vi "_iWorx - Light & Laser.vi"() -> ()   [LabVIEW 2012]
doc: "This VI is designed to work with myDAQ and the iWorx Light Sensor & Laser x2."
uses:
  <vilib>/DAQmx/create/channels.llb/DAQmx Create Channel (AI-Voltage-Basic).vi
  <vilib>/DAQmx/configure/timing.llb/DAQmx Timing (Sample Clock).vi
  <vilib>/DAQmx/read.llb/DAQmx Read (Analog 1D Wfm NChan NSamp).vi
panel:
  in  "Reset Default Cal":bool
  in  "Log Info Button":bool
  in  "Stop":bool
  in  "Threasholds":dbl[](array[numeric])=[1.0, 1.0] format="%.2f V"
  out "Ch 2 Beam Break Duration":dbl format="%.3f s"
  out "Ch 1 Beam Break Duration":dbl format="%.3f s"
  out "Two Edge Seperation":dbl format="%.3f s"
  in  "Set Up":bool
  in  "Pause Button":bool
  in  "Snapshot":bool
  out "Waveform Chart":waveform(dbl)[](graph)
  in  "Clear Chart":bool
  in  "Open Log":bool
  out "Raw Signal":cluster{dbl, dbl}(knob)={0.0, 1.7621809600690803} scale=-5.0..5.0
  # "iWorx - Light Sensor & Laser - Data Logger"
  # "Sensor Input"
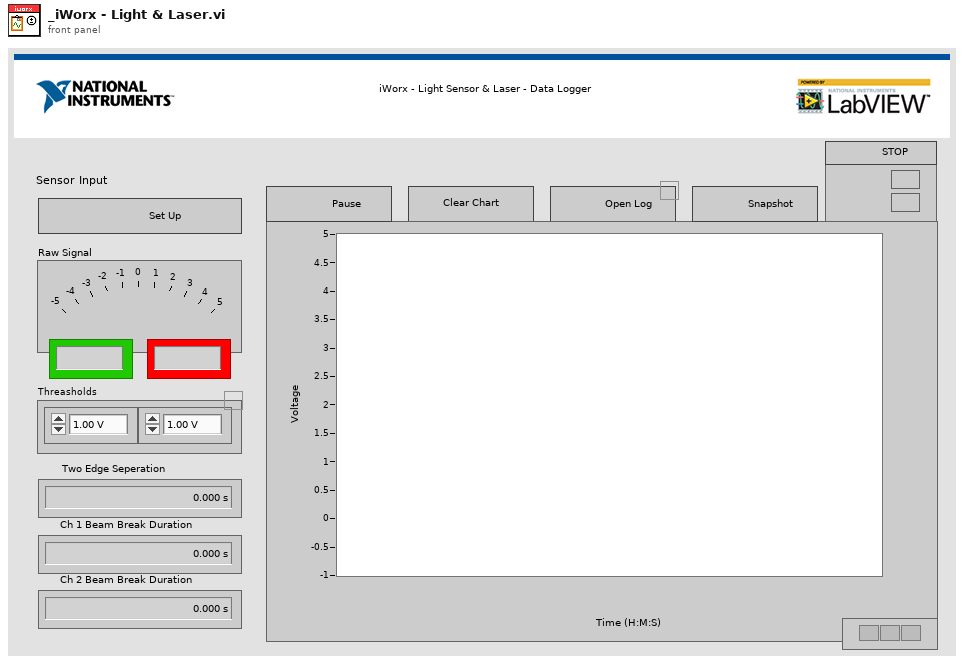
[diagram p1: front panel]
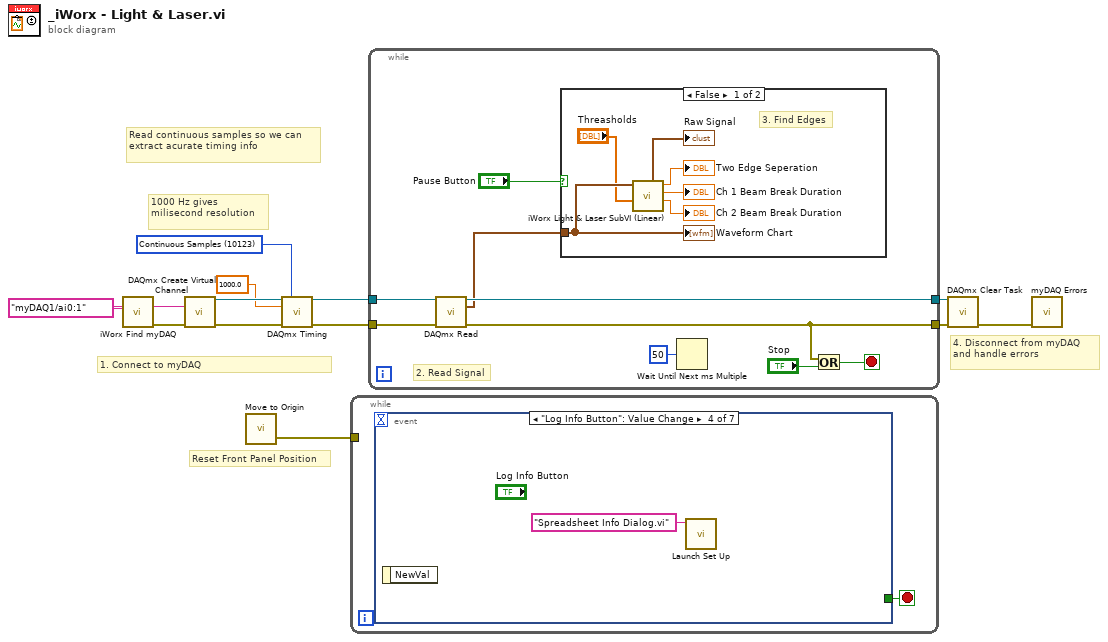
[diagram p0: block diagram]
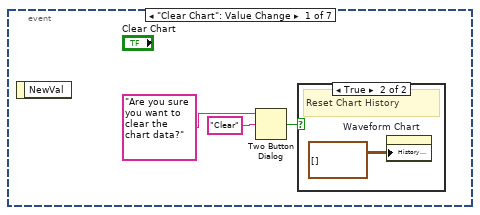
[diagram p2: hidden frame]
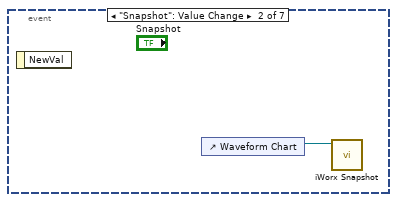
[diagram p4: hidden frame]
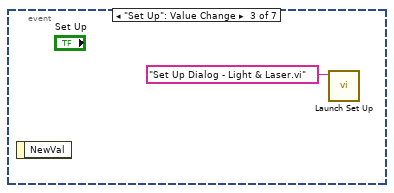
[diagram p5: hidden frame]
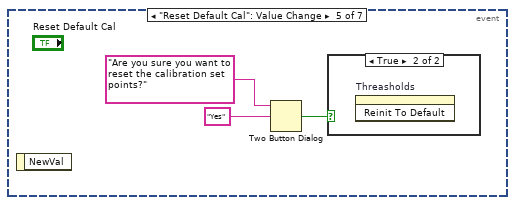
[diagram p6: hidden frame]
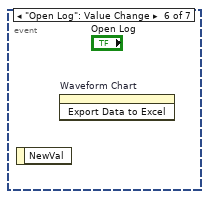
[diagram p8: hidden frame]
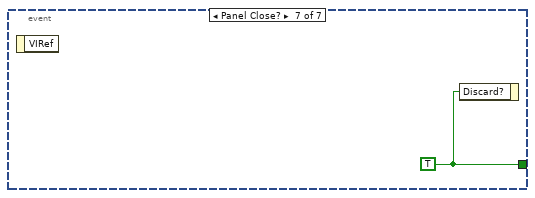
[diagram p9: hidden frame]
diagram:
  w6 = 10123 items=["Finite Samples"=10178, "Continuous Samples"=10123, "Hardware Timed Single Point"=12522] ("sample mode")
  # "Reset Front Panel Position"
  # "4. Disconnect from myDAQ and handle errors"
  # "1. Connect to myDAQ"
  # "1000 Hz gives milisecond resolution"
  # "Read continuous samples so we can extract acurate timing info"
  n1 = call "iWorx Find myDAQ.vi"("Preferred myDAQ (myDAQ1)"=tag "myDAQ1/ai0:1") -> ("Error Out"=w3:errorcluster, "DAQmx Physical Channel"=w4:tag)  [unwired: 6 in, 3 out]
  n2 = call-poly <vilib>:"DAQmx Create Virtual Channel.vi"("physical channels"=w4, "error in"=w3) -> ("task out"=w11:refnum<k21>, "error out"=w8:errorcluster)  [unwired: 12 in]
  n3 = call "Move to Origin.vi"() -> ("Error Out"=w2:errorcluster)  [unwired: 3 in]
  n4 = call-poly <vilib>:"DAQmx Timing.vi"("task/channels in"=w11, "sample mode"=w6, "rate"=1000.0, "error in"=w8) -> ("task out"=w10:refnum<k21>, "error out"=w9:errorcluster)  [unwired: 10 in]
  n5 = while {
    tunnel: w2 -> [_]
    stop <- w14 stop-if-true
    n6 = event shown="[3] \"Log Info Button\": Value Change" {
      selector: _ -> [_ _ _ _ _ _ _]
      dyn-events: _ -> [_ _ _ _ _ _ _]
      timeout: _ -> [_ _ _ _ _ _ _]
      tunnel: [_ _ _ _ _ _ w25] -> w14
      event "Clear Chart": Value Change {
        n7 = event-data() -> ()  [unwired: 1 in, 1 out]
        n8 = Two Button Dialog(message="Are you sure you want to clear the chart data?", 2:"Clear" ("T button name (\"OK\")")) -> (T button?=w16:bool)  [unwired: 1 in]
        n9 = case shown="True" w16 {
          frame False {
            # "Dialog canceled"
          }
          frame True {
            # "Reset Chart History"
            n10 = property on="Waveform Chart" class="WFChart (strict)"("History Data"=waveform(dbl)[][] []) -> ()  [unwired: 2 in, 2 out]
          }
        }
      }
      event "Snapshot": Value Change {
        n11 = event-data() -> ()  [unwired: 1 in, 1 out]
        n12 = control-ref of="Waveform Chart"() -> (w19:refnum<vi>)
        n13 = call "iWorx Snapshot.vi"("WaveformChart in"=w19) -> ()  [unwired: 10 in, 1 out]
      }
      event "Set Up": Value Change {
        n14 = event-data() -> ()  [unwired: 1 in, 1 out]
        n15 = call "Launch Set Up.vi"("name or relative path"="Set Up Dialog - Light & Laser.vi") -> ()  [unwired: 9 in, 2 out]
      }
      event "Log Info Button": Value Change {
        n16 = event-data() -> ()  [unwired: 1 in, 1 out]
        n17 = call "Launch Set Up.vi"("name or relative path"="Spreadsheet Info Dialog.vi") -> ()  [unwired: 9 in, 2 out]
      }
      event "Reset Default Cal": Value Change {
        n18 = event-data() -> ()  [unwired: 1 in, 1 out]
        n19 = Two Button Dialog(message="Are you sure you want to reset the calibration set points?", 2:"Yes" ("T button name (\"OK\")")) -> (T button?=w22:bool)  [unwired: 1 in]
        n20 = case shown="True" w22 {
          frame False {
          }
          frame True {
            n21 = invoke on="Threasholds" class="Arr (strict)" method="Reinit To Default"() -> ()  [unwired: 3 in, 3 out]
          }
        }
      }
      event "Open Log": Value Change {
        n22 = event-data() -> ()  [unwired: 1 in, 1 out]
        n23 = invoke on="Waveform Chart" class="WFChart (strict)" method="Export Data to Excel"() -> ()  [unwired: 3 in, 3 out]
      }
      event Panel Close? {
        w25 = TRUE
        n24 = event-data() -> ()  [unwired: 1 in, 1 out]
        n25 = event-data("Discard?"=w25) -> ()  [unwired: 1 in, 1 out]
      }
    }
  }
  n26 = while {
    tunnel: w10 -> [w34]
    tunnel: [w29] -> w13
    tunnel: w9 -> [w33]
    tunnel: [w31] -> w12
    stop <- w32 stop-if-true
    # "2. Read Signal"
    n27 = call-poly <vilib>:"DAQmx Read.vi"("task/channels in"=w34, "error in"=w33) -> ("task out"=w29:refnum<k21>, "data"=w28:waveform(dbl)[], "error out"=w31:errorcluster)  [unwired: 11 in]
    n28 = case shown="False" "Pause Button" {
      tunnel: w28 -> [w36 _]
      frame False {
        # "3. Find Edges"
        n29 = call "iWorx Light & Laser SubVI (Linear).vi"("Threasholds (1V)"="Threasholds", "Waveform Array"=w36) -> ("Ch 2 Beam Break Duration (s)"=→"Ch 2 Beam Break Duration":dbl, "Ch 1 Beam Break Duration (s)"=→"Ch 1 Beam Break Duration":dbl, "Two Edge Seperation (s)"=→"Two Edge Seperation":dbl, "Raw Signal"=→"Raw Signal":cluster{dbl, dbl})  [unwired: 5 in, 1 out]
        "Waveform Chart" <- w36
      }
      frame True {
      }
    }
    n30 = Wait Until Next ms Multiple(millisecond multiple=u32 50) -> ()  [unwired: 1 out]
    n31 = Or(x=w31, y="Stop") -> (x .or. y?=w32:bool)
  }
  n32 = call <vilib>:"DAQmx Clear Task.vi"("task in"=w13, "error in"=w12) -> ("error out"=w1:errorcluster)  [unwired: 13 in]
  n33 = call "myDAQ Errors.vi"("error in (no error)"=w1) -> ()  [unwired: 10 in, 1 out]
